vi "JSON to LVObject - Object With Member And JSON Object With Member - Returns Same Object With Member Set.vi"() -> ()   [LabVIEW 2017, in "Generic Object Serializer Tests.lvlib"]
uses:
  Generic Object Serializer Tests.lvlib
  Generic Object Serializer/Generic Object Serializer.lvclass
  Weather Forecast/Weather Forecast.lvclass
  <vilib>/addons/_JKI Toolkits/Caraya/classes/Assert/Assert Equal Value and Type_Variant.vi
  <vilib>/addons/_JKI Toolkits/Caraya/classes/Test/Test.lvclass
  <vilib>/addons/_JKI Toolkits/Caraya/classes/Assert/Assert.lvclass
panel:
  out "error out":errorcluster
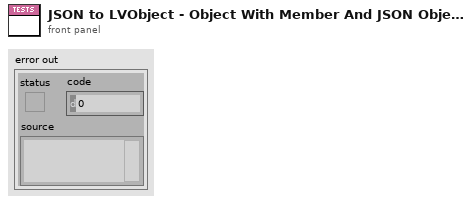
[diagram p1: front panel]
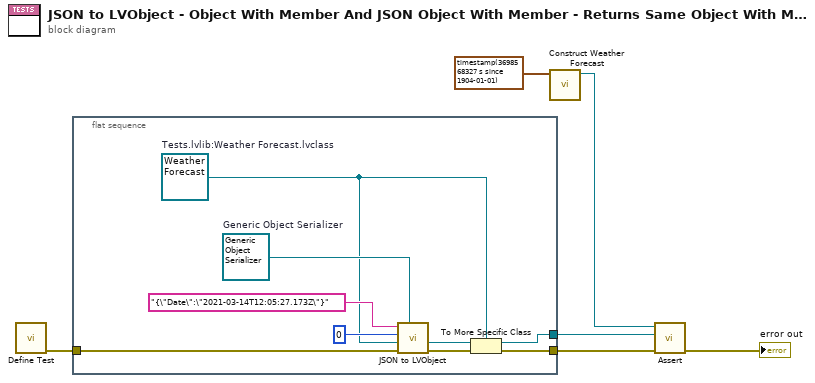
[diagram p0: block diagram]
diagram:
  n1 = call <vilib>:"Define Test.vi"() -> ("error out"=w6:errorcluster)  [unwired: 11 in]
  n2 = flat-sequence {
    tunnel: w6 -> [w14]
    tunnel: [w10] -> w5
    tunnel: [w7] -> w4
    frame #0 {
      w8 = refnum<class "Weather Forecast.lvclass"> refnum  # Tests.lvlib:Weather Forecast.lvclass
      w15 = refnum<class "Generic Object Serializer.lvclass"> refnum  # Generic Object Serializer
      n3 = call-dynamic "JSON to LVObject.vi"("LVClass Serializer"=w15, "error in (no error)"=w14, "Object Type"=w8, "Offset"=0, "JSON"="{\"Date\":\"2021-03-14T12:05:27.173Z\"}") -> ("error out"=w13:errorcluster, "Object"=w9:refnum<class>)  [unwired: 5 in]
      n4 = To More Specific Class(target class=w8, reference=w9, error in=w13) -> (specific class reference=w7:refnum<class "Weather Forecast.lvclass">, error out=w10:errorcluster)
    }
  }
  n5 = call "Construct Weather Forecast.vi"("Date"=timestamp(3698568327.173 s since 1904-01-01)) -> ("Weather Forecast"=w2:refnum<class "Weather Forecast.lvclass">)  [unwired: 9 in, 1 out]
  n6 = call-poly <vilib>:"Assert.vi"("error in (no error)"=w5, "Y"=w4, "X"=w2) -> ("error out"=→"error out":errorcluster)  [unwired: 8 in]
